vi "PV Integrated Pressure Sensors.vi"(8 "error in (no error)":errorcluster, 9 "PV Integrated pressure Sensor - Cluster":T1={"Parameter"=enum." Pressure 1 value [hPa] (740) (default)", "Parameter\nread only<->describe"=FALSE, "Correction facktor\n(0,20 - 9,90) "=1.0, "Pressure set point (hPa)\n0 => ur (p<1,0e-5 hPa)\n850 - 1250 hPa"=0, "Pressure switch\npoint (hPa)"=1.0, "Pressure HV enable (IKT010 only)"=0} {"Pressure HV enable (IKT010 only)" items=["off", "on", "on above TMP speed switchpoint", "on below pressure 2 switchpoint"]; "Pressure switch\npoint (hPa)" min=5e-10 max=2000.0 step=1.0 format="%_3e"; "Pressure set point (hPa)\n0 => ur (p<1,0e-5 hPa)\n850 - 1250 hPa" min=0 max=2050 step=1; "Correction facktor\n(0,20 - 9,90)" min=0.2 max=9.9 step=0.01 format="%.2f"}, 10 "Adress of unit":u16=1 min=1 max=999 step=1, 11 "VISA session":refnum<visa-resource-name>) -> (0 "error out":errorcluster, 2 "response (data)":string, 3 "dup VISA session":refnum<visa-resource-name>)   [LabVIEW 2021, in "Pfeiffer Vacuum.lvlib"]
doc: "There are 9 parameters available, only one of which can be enabled at a time. \n\n0 - Pressure 1 switchpoint [hPa] (730) (default)\n1 - Pressure 2 switchpoint [hPa] (732)\n2 - Name of sensor 1 (739)\n3 - Pressure 1 value [hPa] (740)\n4 - Correction factor 1 (742)\n5 - Name of sensor 2 (749)\n6 - Pressure 2 value [hPa] (750)\n7 - Correction factor 2 (752)\n8 - Pressure HV enable (IKT010 only) (041)\n\nNote: Any settings for an parameter that is not selected will be ignored. If a value is out of range, it will be changed to either the upper or the lower limit of the range."
uses:
  <instrlib>/Pfeiffer Vacuum/Pfeiffer Vacuum.lvlib
  <instrlib>/Pfeiffer Vacuum/Public/Turbopumps/PV Integrated Pressure Sensors - Cluster.ctl
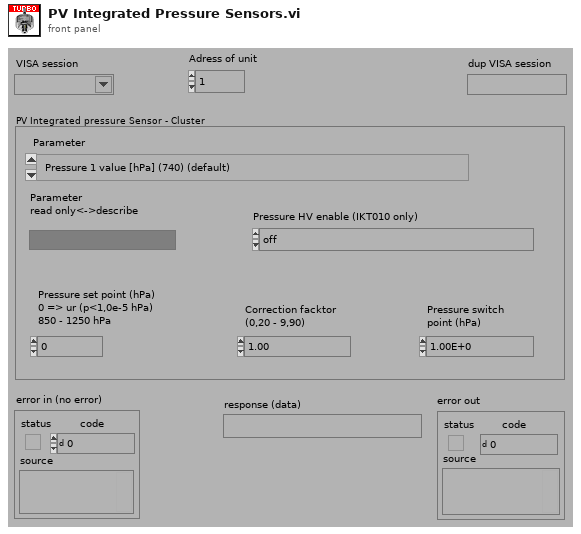
[diagram p1: front panel]
types:
  T1 = typedef "Pfeiffer Vacuum.lvlib/PV Integrated Pressure Sensors - Cluster.ctl" = cluster{"Parameter":enum16{" Pressure 1 switchpoint [hPa] (730) (default)", " Pressure 2 switchpoint [hPa] (732)", " Name of sensor 1 (739)", " Pressure 1 value [hPa] (740) (default)", " Correction factor 1 (742)", " Name of sensor 2 (749)", " Pressure 2 value [hPa] (750)", " Correction factor 2 (752)", " Pressure HV enable (IKT010 only) (041)"}, "Parameter\nread only<->describe":bool, "Correction facktor\n(0,20 - 9,90) ":sgl, "Pressure set point (hPa)\n0 => ur (p<1,0e-5 hPa)\n850 - 1250 hPa":i16, "Pressure switch\npoint (hPa)":dbl, "Pressure HV enable (IKT010 only)":u16}
  T2 = enum16{" Pressure 1 switchpoint [hPa] (730) (default)", " Pressure 2 switchpoint [hPa] (732)", " Name of sensor 1 (739)", " Pressure 1 value [hPa] (740) (default)", " Correction factor 1 (742)", " Name of sensor 2 (749)", " Pressure 2 value [hPa] (750)", " Correction factor 2 (752)", " Pressure HV enable (IKT010 only) (041)"}
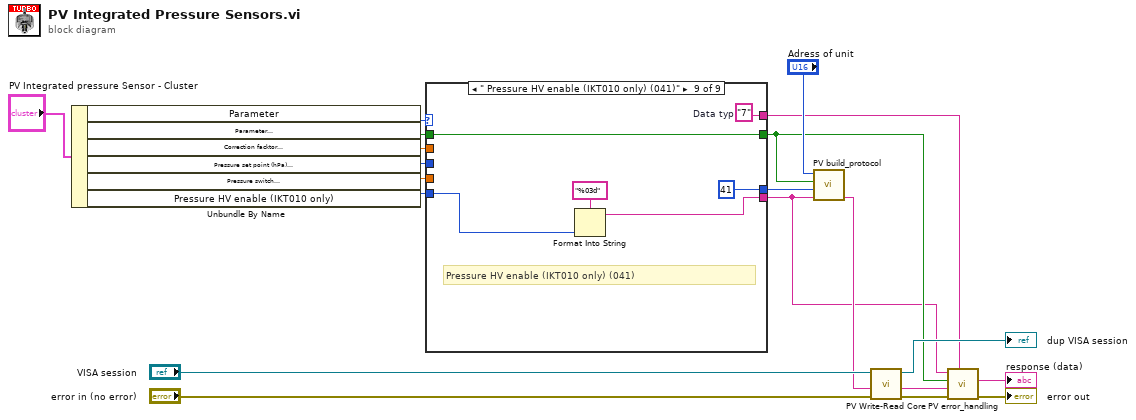
[diagram p0: block diagram]
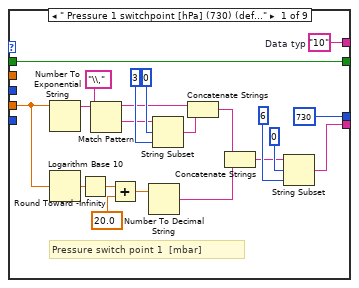
[diagram p2: hidden frame]
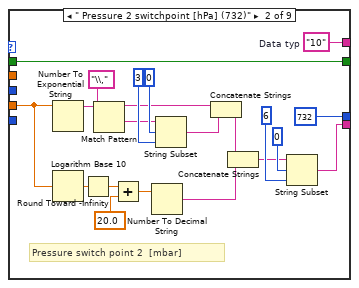
[diagram p3: hidden frame]
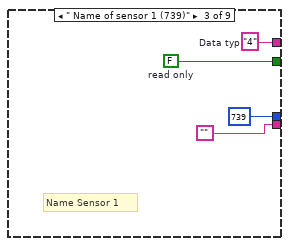
[diagram p4: hidden frame]
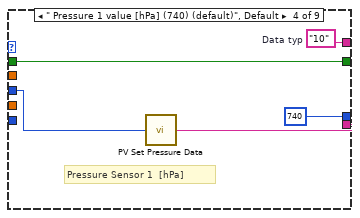
[diagram p5: hidden frame]
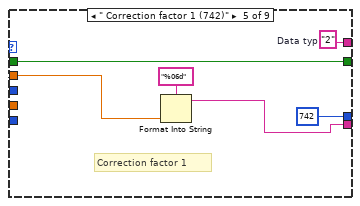
[diagram p6: hidden frame]
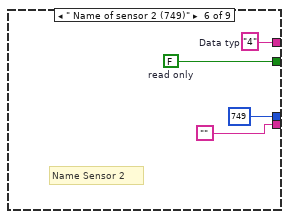
[diagram p7: hidden frame]
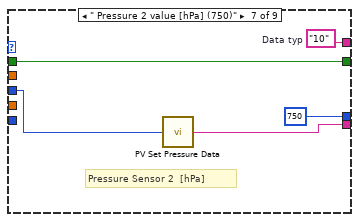
[diagram p8: hidden frame]
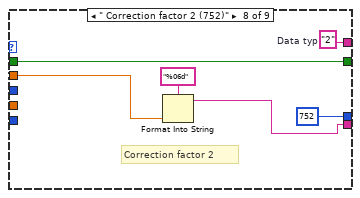
[diagram p9: hidden frame]
diagram:
  n1 = Unbundle By Name("PV Integrated pressure Sensor - Cluster") -> ("Parameter"=w18:T2, "Parameter\nread only<->describe"=w17:bool, "Correction facktor\n(0,20 - 9,90)"=w5:sgl, "Pressure set point (hPa)\n0 => ur (p<1,0e-5 hPa)\n850 - 1250 hPa"=w4:i16, "Pressure switch\npoint (hPa)"=w3:dbl, "Pressure HV enable (IKT010 only)"=w2:u16)
  n2 = case shown="\" Pressure HV enable (IKT010 only) (041)\"" w18 {
    tunnel: [u16 730 ("Parameter-number") u16 732 ("Parameter-number") u16 739 ("Parameter-number") u16 740 ("Parameter-number") u16 742 ("Parameter-number") u16 749 ("Parameter-number") u16 750 ("Parameter-number") u16 752 ("Parameter-number") u16 41 ("Parameter-number")] -> w19
    tunnel: [w22 w43 "" w67 w74 "" w83 w90 w96] -> w9
    tunnel: [w40 w61 w64 w69 w73 w80 w85 w89 w99] -> w10
    tunnel: w17 -> [w40 w61 _ w69 w73 _ w85 w89 w99]
    tunnel: [w39 w60 w65 w70 w77 w81 w86 w93 w101] -> w8
    tunnel: w5 -> [_ _ _ _ w72 _ _ w88 w98]
    tunnel: w4 -> [_ _ _ w68 _ _ w84 _ _]
    tunnel: w3 -> [w21 w42 _ _ _ _ _ _ _]
    tunnel: w2 -> [_ _ _ _ _ _ _ _ w95]
    frame " Pressure 1 switchpoint [hPa] (730) (default)" {
      w39 = "10"  # Data typ
      # "Pressure switch point 1  [mbar]"
      n3 = Number To Exponential String(number=w21) -> (E-format string=w27:string)  [unwired: 3 in]
      n4 = Logarithm Base 10(1:w21) -> (0:w23:dbl)
      n5 = Round Toward -Infinity(1:w23) -> (0:w24:dbl)
      n6 = Match Pattern(string=w27, regular expression="\\,") -> (before substring=w26:string, after substring=w28:string)  [unwired: 1 in, 2 out]
      n7 = Add(x=w24, y=20.0) -> (x+y=w32:dbl)
      n8 = Number To Decimal String(number=w32) -> (decimal integer string=w35:string)  [unwired: 1 in]
      n9 = String Subset(string=w28, offset (0)=0 ("Offset (0)"), length (rest)=3 ("Länge")) -> (substring=w31:string)
      n10 = Concatenate Strings(w26, w31) -> (w34:string)
      n11 = Concatenate Strings(w34, w35) -> (w36:string)
      n12 = String Subset(string=w36, offset (0)=0 ("Offset (0)"), length (rest)=6 ("Länge")) -> (substring=w22:string)
    }
    frame " Pressure 2 switchpoint [hPa] (732)" {
      w60 = "10"  # Data typ
      # "Pressure switch point 2  [mbar]"
      n13 = Number To Exponential String(number=w42) -> (E-format string=w48:string)  [unwired: 3 in]
      n14 = Logarithm Base 10(1:w42) -> (0:w44:dbl)
      n15 = Round Toward -Infinity(1:w44) -> (0:w45:dbl)
      n16 = Match Pattern(string=w48, regular expression="\\,") -> (before substring=w47:string, after substring=w49:string)  [unwired: 1 in, 2 out]
      n17 = Add(x=w45, y=20.0) -> (x+y=w53:dbl)
      n18 = Number To Decimal String(number=w53) -> (decimal integer string=w56:string)  [unwired: 1 in]
      n19 = String Subset(string=w49, offset (0)=0 ("Offset (0)"), length (rest)=3 ("Länge")) -> (substring=w52:string)
      n20 = Concatenate Strings(w47, w52) -> (w55:string)
      n21 = Concatenate Strings(w55, w56) -> (w57:string)
      n22 = String Subset(string=w57, offset (0)=0 ("Offset (0)"), length (rest)=6 ("Länge")) -> (substring=w43:string)
    }
    frame " Name of sensor 1 (739)" {
      w64 = FALSE  # read only
      w65 = "4"  # Data typ
      # "Name Sensor 1"
    }
    frame " Pressure 1 value [hPa] (740) (default)", Default {
      w70 = "10"  # Data typ
      # "Pressure Sensor 1  [hPa]"
      n23 = call <instrlib>:"PV Set Pressure Data.vi"("Pressure (mbar)\n0 ==> ur (<1,0e-4mbar)\n1 - 2050 mbar"=w68) -> ("Output"=w67:string)
    }
    frame " Correction factor 1 (742)" {
      w77 = "2"  # Data typ
      # "Correction factor 1"
      n24 = Multiply(x=w72, y=100.0) -> ()  [unwired: 1 out]
      n25 = Format Into String(format string="%06d" ("Format-String"), w72) -> (resulting string=w74:string)  [unwired: 2 in, 1 out]
    }
    frame " Name of sensor 2 (749)" {
      w80 = FALSE  # read only
      w81 = "4"  # Data typ
      # "Name Sensor 2"
    }
    frame " Pressure 2 value [hPa] (750)" {
      w86 = "10"  # Data typ
      # "Pressure Sensor 2  [hPa]"
      n26 = call <instrlib>:"PV Set Pressure Data.vi"("Pressure (mbar)\n0 ==> ur (<1,0e-4mbar)\n1 - 2050 mbar"=w84) -> ("Output"=w83:string)
    }
    frame " Correction factor 2 (752)" {
      w93 = "2"  # Data typ
      # "Correction factor 2"
      n27 = Multiply(x=w88, y=100.0) -> ()  [unwired: 1 out]
      n28 = Format Into String(format string="%06d" ("Format-String"), w88) -> (resulting string=w90:string)  [unwired: 2 in, 1 out]
    }
    frame " Pressure HV enable (IKT010 only) (041)" {
      w101 = "7"  # Data typ
      # "Pressure HV enable (IKT010 only) (041)"
      n29 = Multiply(x=w98, y=100.0) -> ()  [unwired: 1 out]
      n30 = Format Into String(format string="%03d" ("Format-String"), w95) -> (resulting string=w96:string)  [unwired: 2 in, 1 out]
    }
  }
  n31 = call <instrlib>:"PV build_protocol.vi"("Data"=w9, "Parameter-number"=w19, "parameter\nread<->describe"=w10, "Adress"="Adress of unit") -> ("output"=w14:string)  [unwired: 3 in]
  n32 = call <instrlib>:"PV Write-Read Core.vi"("error in"="error in (no error)", "Write data in"=w14, "VISA session"="VISA session") -> ("error out"=w11:errorcluster, "response (data) out"=w12:string, "dup VISA session"=→"dup VISA session":refnum<visa-resource-name>)  [unwired: 2 in]
  n33 = call <instrlib>:"PV error_handling.vi"("Data Typ in"=w8, "error in"=w11, "response (data) in"=w12, "Parameter\nread only<->describe"=w10, "data in"=w9) -> ("error out"=→"error out":errorcluster, "Data out"=→"response (data)":string)  [unwired: 4 in, 1 out]
